vi "GEN40-38-LAN Send Output Setting.vi"(8 "error in (no error)":errorcluster, 11 "GEN40-38-LAN in":refnum<class "GEN40-38-LAN.lvclass">) -> (0 "error out":errorcluster, 3 "GEN40-38-LAN out":refnum<class "GEN40-38-LAN.lvclass">)   [LabVIEW 2018, in "GEN40-38-LAN.lvlib" / "GEN40-38-LAN.lvclass"]
doc: "This VI is used to send the output setting to the Power Supply."
uses:
  GEN40-38-LAN.lvclass
  PPLs/Power Supply/Parent/Power_Supply.lvlibp/Power Supply.lvclass
  C:/Projects/LabVIEW/PPLs/Power Supply/Parent/Power_Supply.lvlibp/Power Supply.lvclass
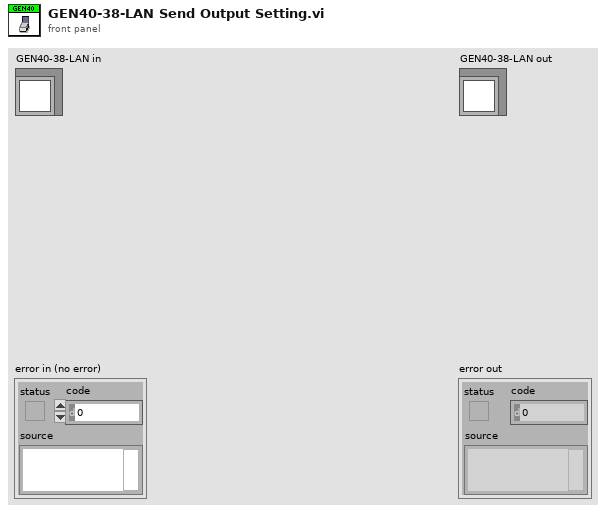
[diagram p1: front panel]
types:
  T1 = typedef "Power_Supply.lvlibp/Supply Settings.ctl" = cluster{"Voltage":dbl, "Current":dbl, "Output":bool}
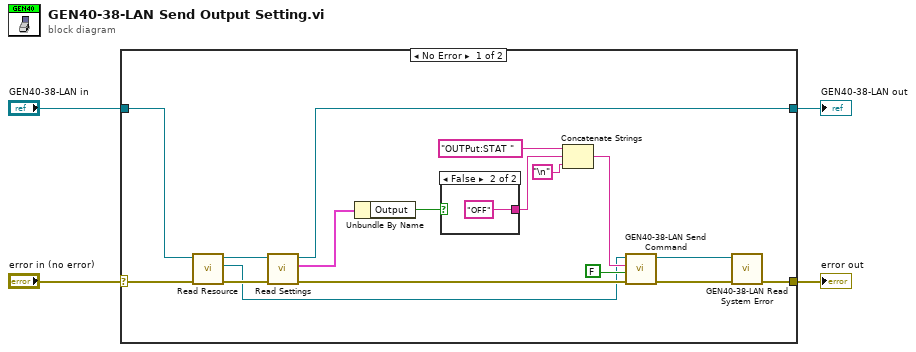
[diagram p0: block diagram]
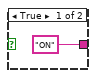
[diagram p2: hidden frame]
diagram:
  n1 = case shown="No Error" "error in (no error)" {
    selector: "error in (no error)" -> [w20 w25]
    tunnel: [w5 w25] -> w4
    tunnel: [w16 w24] -> w2
    tunnel: "GEN40-38-LAN in" -> [w21 w24]
    frame No Error {
      n2 = call "Read Resource.vi"("error in"=w20, "Power Supply in"=w21) -> ("error out"=w19:errorcluster, "Resource"=w8:refnum<visa-resource-name>, "Power Supply out"=w18:refnum<class "GEN40-38-LAN.lvclass">)  [unwired: 7 in]
      n3 = call "Read Settings.vi"("error in (no error)"=w19, "Power Supply in"=w18) -> ("error out"=w11:errorcluster, "Settings"=w17:T1, "Power Supply out"=w16:refnum<class "GEN40-38-LAN.lvclass">)  [unwired: 7 in]
      n4 = Unbundle By Name(w17) -> ("Output"=w10:bool)
      n5 = case shown="False" w10 {
        tunnel: ["ON" "OFF"] -> w9
        frame True {
        }
        frame False {
        }
      }
      n6 = Concatenate Strings("OUTPut:STAT ", w9, "\n" ("string")) -> (w13:string)
      n7 = call "GEN40-38-LAN Send Command.vi"("error in (no error)"=w11, "Wait for Response?"=FALSE, "Command"=w13, "VISA resource name"=w8) -> ("error out"=w6:errorcluster, "VISA resource name out"=w7:refnum<visa-resource-name>)  [unwired: 5 in, 1 out]
      n8 = call "GEN40-38-LAN Read System Error.vi"("error in (no error)"=w6, "Resource"=w7) -> ("error out"=w5:errorcluster)  [unwired: 9 in]
    }
    frame Error {
    }
  }
  "error out" <- w4
  "GEN40-38-LAN out" <- w2
